vi "Update Run Parameters.vi"(8 "error in (no error)":errorcluster, 10 "Parameters":string[][](array[string]), 11 "Optimiser Cell in":refnum<class "Schedule Cell.lvclass">) -> (0 "error out":errorcluster, 3 "Optimiser Cell out":refnum<class "Schedule Cell.lvclass">)   [LabVIEW 2020, in "Run Utilities.lvlib" / "Schedule Cell.lvclass"]
doc: "Update parameters of the Run Instance inside the cell. It will only modify existing parameters"
uses:
  Schedule Cell.lvclass
  Schedule Cell.lvclass/Schedule Cell.ctl
  Run Instance/Run Instance.lvclass
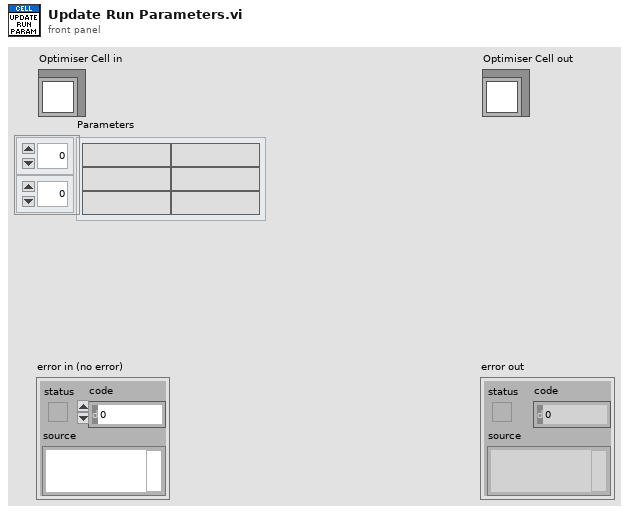
[diagram p1: front panel]
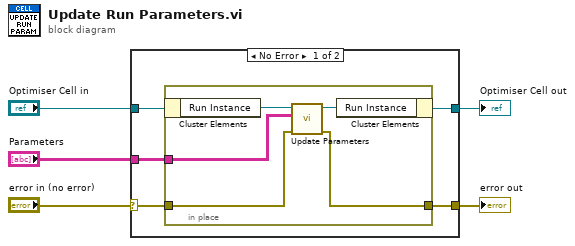
[diagram p0: block diagram]
diagram:
  n1 = case shown="No Error" "error in (no error)" {
    selector: "error in (no error)" -> [w7 w17]
    tunnel: [w6 w17] -> w4
    tunnel: [w9 w16] -> w2
    tunnel: "Optimiser Cell in" -> [w10 w16]
    tunnel: "Parameters" -> [w8 _]
    frame No Error {
      n2 = in-place {
        in-place-border: w8 -> [w13]
        in-place-border: w7 -> [w12]
        in-place-border: [w11] -> w6
        n3 = in-place-cluster #1(w10) -> ("Run Instance"=w14:refnum<class "Run Instance.lvclass">)
        n4 = call-dynamic "Update Parameters.vi"("error in (no error)"=w12, "Parameters"=w13, "Run Instance in"=w14) -> ("error out"=w11:errorcluster, "Run Instance out"=w15:refnum<class "Run Instance.lvclass">)  [unwired: 6 in, 1 out]
        n5 = in-place-cluster #1("Run Instance"=w15) -> (w9:refnum<class "Schedule Cell.lvclass">)
      }
    }
    frame Error {
    }
  }
  "error out" <- w4
  "Optimiser Cell out" <- w2
